vi "Crab Drive.vi"(10 "Joy Y":dbl, 11 "Joy X":dbl) -> (2 "Speed":dbl, 3 "Wheel Angle":dbl)   [LabVIEW 2011]
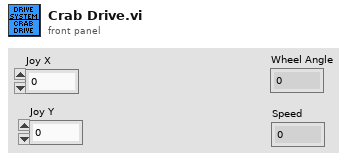
[diagram p1: front panel]
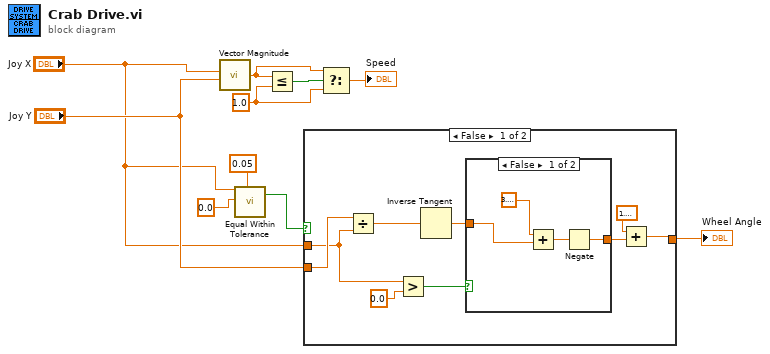
[diagram p0: block diagram]
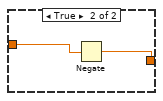
[diagram p2: hidden frame]
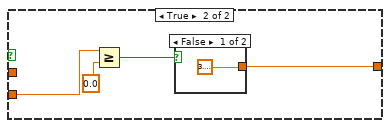
[diagram p3: hidden frame]
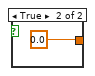
[diagram p4: hidden frame]
diagram:
  w9 = 1.0 ("y")
  n1 = call "Vector Magnitude.vi"("X Component"="Joy X", "Y Component"="Joy Y") -> ("Magnitude"=w8:dbl)  [unwired: 6 in]
  n2 = call "Equal Within Tolerance.vi"("Number In"="Joy X", "Comparison Value"=0.0, "Tolerance"=0.05) -> ("Equality"=w5:bool)  [unwired: 16 in]
  n3 = Less Or Equal?(x=w8, y=w9) -> (x <= y?=w10:bool)
  n4 = case shown="False" w5 {
    tunnel: "Joy Y" -> [w19 w29]
    tunnel: [w12 w26] -> w3
    tunnel: "Joy X" -> [w16 _]
    frame False {
      n5 = Divide(x=w19, y=w16) -> (x/y=w18:dbl)
      n6 = Greater?(x=w16, y=0.0) -> (0:w14:bool)
      n7 = Inverse Tangent(1:w18) -> (0:w17:dbl)
      n8 = case shown="False" w14 {
        tunnel: w17 -> [w23 w25]
        tunnel: [w21 w24] -> w13
        frame False {
          n9 = Add(x=3.141592653589793, y=w23) -> (x+y=w22:dbl)
          n10 = Negate(x=w22) -> (-x=w21:dbl)
        }
        frame True {
          n11 = Negate(x=w25) -> (-x=w24:dbl)
        }
      }
      n12 = Add(x=1.5707963267948966, y=w13) -> (x+y=w12:dbl)
    }
    frame True {
      n13 = Greater Or Equal?(x=w29, y=0.0) -> (x >= y?=w27:bool)
      n14 = case shown="False" w27 {
        tunnel: [3.141592653589793 0.0 ("y")] -> w26
        frame False {
        }
        frame True {
        }
      }
    }
  }
  "Wheel Angle" <- w3
  n15 = Select(t=w8, s=w10, f=w9) -> (s? t:f=→"Speed":dbl)
